vi "error_handler.vi"(8 "error in (no error)":errorcluster, 11 "manager_daemon in":refnum<class "manager_daemon.lvclass">) -> (0 "error out":errorcluster, 3 "manager_daemon out":refnum<class "manager_daemon.lvclass">)   [LabVIEW 2024, in "manager_daemon.lvclass"]
uses:
  manager_daemon.lvclass
  manager_daemon.lvclass/manager_daemon.ctl
  type_defs/cmd--enum.ctl
  type_defs/msg--cluster.ctl
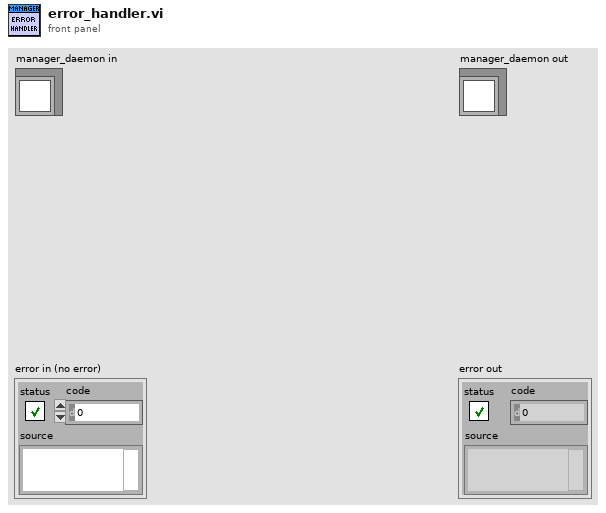
[diagram p1: front panel]
types:
  T1 = typedef "manager_daemon.lvclass/msg--cluster.ctl" = cluster{"cmd":T2, "data":variant}
  T2 = typedef "manager_daemon.lvclass/cmd--enum.ctl" = enum16{"init", "run", "load binaries", "build binaries", "save binaries", "updated volume", "return vol path by id", "display info", "filter release week", "apply filter", "add publisher", "get publishers", "add volume", "add issues", "add issue", "delete volume", "delete issues", "download issues", "exit"}
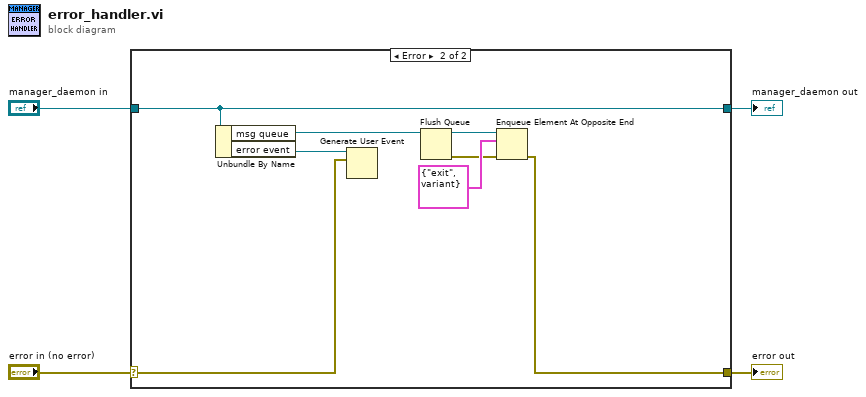
[diagram p0: block diagram]
diagram:
  n1 = case shown="Error" "error in (no error)" {
    selector: "error in (no error)" -> [w5 w12]
    tunnel: [w5 w7] -> w3
    tunnel: [w6 w14] -> w1
    tunnel: "manager_daemon in" -> [w6 w14]
    frame No Error {
    }
    frame Error {
      n2 = Unbundle By Name(w14) -> ("msg queue"=w11:refnum<queue>, "error event"=w13:refnum<user-event>)
      n3 = Generate User Event(user event=w13, event data cluster=w12) -> ()  [unwired: 2 in, 2 out]
      n4 = Flush Queue(queue=w11) -> (queue out=w10:refnum<queue>, error out=w8:errorcluster)  [unwired: 1 in, 1 out]
      n5 = Enqueue Element At Opposite End(queue=w10, element=T1 {"cmd"=enum."exit", "data"=variant}, error in (no error)=w8) -> (error out=w7:errorcluster)  [unwired: 1 in, 2 out]
    }
  }
  "error out" <- w3
  "manager_daemon out" <- w1
